vi "Load_Sequence.vi"(8 "error in (no error)":errorcluster, 9 "operation (0:open)":T4(ring), 10 "relative Path":bool, 11 "Path":path=path "Seq-03.csv") -> (0 "error out":errorcluster, 2 "General_Info":T1, 3 "Seq_Measurement":T3(array[cluster]))   [LabVIEW 2023]
panel:
  in  "Sequnce_Info":T2
  out "Edit_Seq_Array_Output":T3(array[cluster])
  in  "Edit_Seq_Array_Input":T3(array[cluster]) {"THD_Limit" min=0.0 max=1.0 step=0.01; "Noise" min=0.0 max=10.0 step=0.1; "Frequency" min=0.0 max=1000.0 step=1.0; "Amplitude" min=0.0 max=10.0 step=0.1}
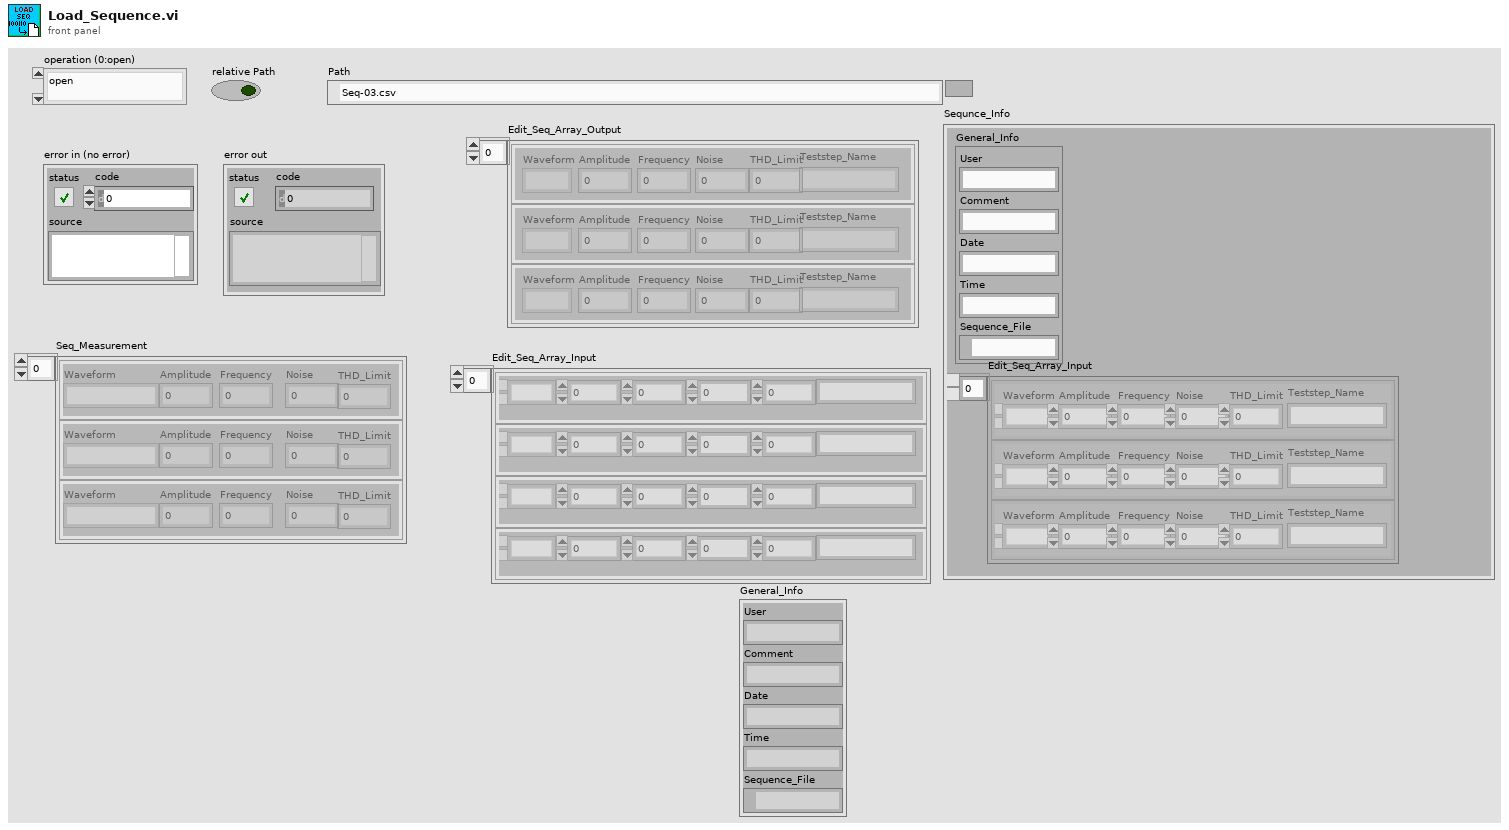
[diagram p1: front panel]
types:
  T1 = cluster{"User":string, "Comment":string, "Date":string, "Time":string, "Sequence_File":path}
  T2 = cluster{"General_Info":cluster{"User":string, "Comment":string, "Date":string, "Time":string, "Sequence_File":path}, "Edit_Seq_Array_Input":cluster{"Waveform":enum16{"", "Sine Wave", "Triangle Wave", "Square Wave", "Sawtooth Wave"}, "Amplitude":dbl, "Frequency":dbl, "Noise":dbl, "THD_Limit":dbl, "Teststep_Name":string}[]}
  T3 = cluster{"Waveform":enum16{"", "Sine Wave", "Triangle Wave", "Square Wave", "Sawtooth Wave"}, "Amplitude":dbl, "Frequency":dbl, "Noise":dbl, "THD_Limit":dbl, "Teststep_Name":string}[]
  T4 = enum16{"open", "replace", "create", "open or create", "replace or create", "replace or create with confirmation"}
  T5 = enum16{"", "Sine Wave", "Triangle Wave", "Square Wave", "Sawtooth Wave"}
  T6 = cluster{"Waveform":enum16{"", "Sine Wave", "Triangle Wave", "Square Wave", "Sawtooth Wave"}, "Amplitude":dbl, "Frequency":dbl, "Noise":dbl, "THD_Limit":dbl, "Teststep_Name":string}
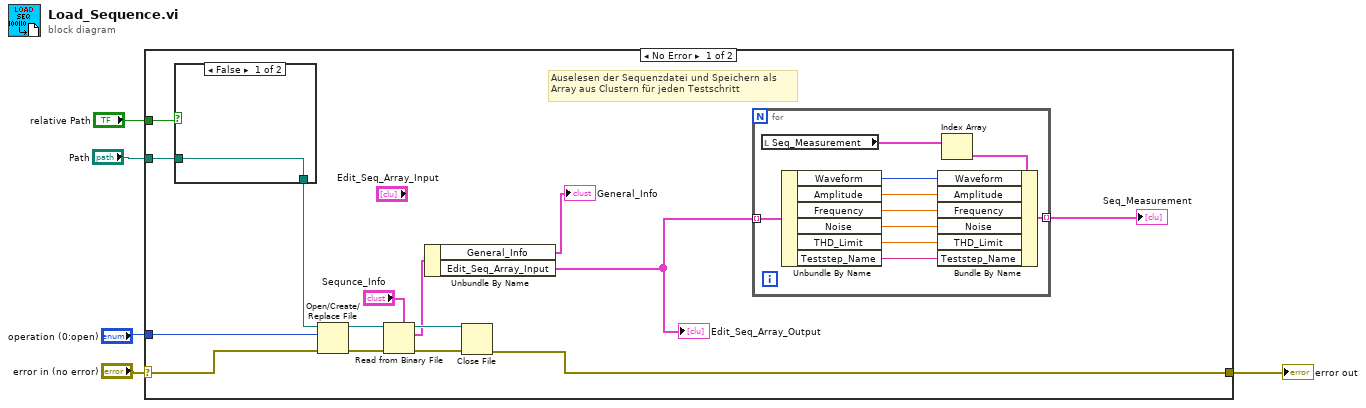
[diagram p0: block diagram]
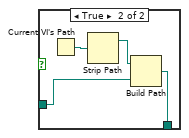
[diagram p2: hidden frame]
diagram:
  n1 = case shown="No Error" "error in (no error)" {
    selector: "error in (no error)" -> [w20 w36]
    tunnel: [w17 w36] -> w5
    tunnel: "Path" -> [w12 _]
    tunnel: "operation (0:open)" -> [w13 _]
    tunnel: "relative Path" -> [w10 _]
    frame No Error {
      # "Auselesen der Sequenzdatei und Speichern als \nArray aus Clustern für jeden Testschritt"
      n2 = case shown="False" w10 {
        tunnel: w12 -> [w21 w23]
        tunnel: [w21 w22] -> w11
        frame False {
        }
        frame True {
          n3 = Current VI's Path() -> (path=w25:path)
          n4 = Strip Path(path=w25) -> (stripped path=w24:path)  [unwired: 1 out]
          n5 = Build Path(base path=w24, name or relative path=w23) -> (appended path=w22:path)
        }
      }
      n6 = Open/Create/Replace File(file path (use dialog)=w11, error in=w20, operation (0:open)=w13) -> (refnum out=w16:refnum<file>, error out=w19:errorcluster)  [unwired: 3 in, 1 out]
      n7 = Read from Binary File(5:"Sequnce_Info", 8:w19, 11:w16) -> (0:w18:errorcluster, 2:w8:T2, 3:w15:refnum<file>)  [unwired: 3 in, 1 out]
      n8 = Unbundle By Name(w8) -> ("General_Info"=→"General_Info":T1, "Edit_Seq_Array_Input"=w7:T3)
      "Edit_Seq_Array_Output" <- w7
      n9 = Close File(refnum=w15, error in=w18) -> (error out=w17:errorcluster)  [unwired: 1 out]
      n10 = for {
        tunnel: w7 -> [w35] mode=indexing
        tunnel: [w27] -> w14 mode=indexing
        n11 = local read "Seq_Measurement"() -> (w29:T3)
        n12 = Unbundle By Name(w35) -> ("Waveform"=w34:T5, "Amplitude"=w33:dbl, "Frequency"=w32:dbl, "Noise"=w31:dbl, "THD_Limit"=w30:dbl, "Teststep_Name"=w26:string)
        n13 = Index Array(array=w29) -> (element=w28:T6)  [unwired: 1 in]
        n14 = Bundle By Name(cluster=w28, "Waveform"=w34, "Amplitude"=w33, "Frequency"=w32, "Noise"=w31, "THD_Limit"=w30, "Teststep_Name"=w26) -> (w27:T6)
      }
      "Seq_Measurement" <- w14
    }
    frame Error {
    }
  }
  "error out" <- w5
